vi "Main.vi"() -> ()   [LabVIEW 2018, in "Personalities Tool.lvlib"]
uses:
  Personalities Tool.lvlib
  Controls/QMH Data.ctl
  Controls/Personality Type.ctl
  Controls/roboRIO Connection Information.ctl
  Controls/Diff Key.ctl
  subVIs/Message Queue/Enqueue Message (Single).vi
panel:
  out "Personality":string
  out "Status":string
  in  "File editor":string
  in  "Download personality to RIO":bool
  in  "Save personality locally":bool
  in  "Connect":bool
  in  "Open local personality":bool
  in  "Stop":bool
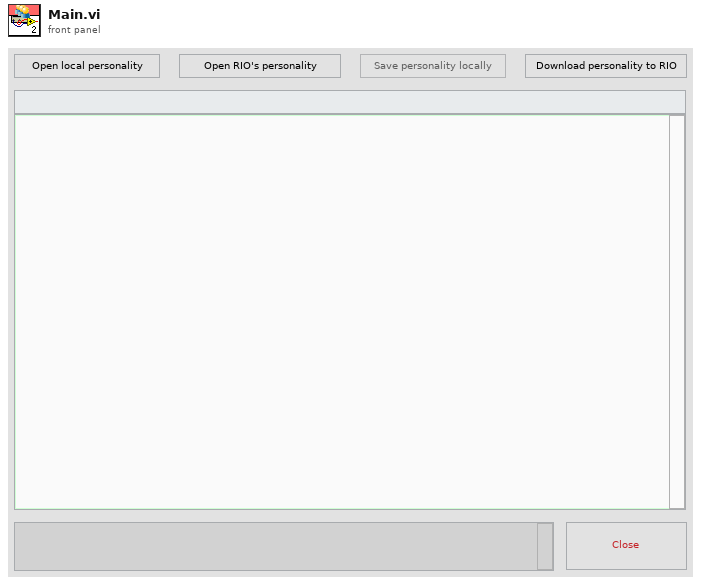
[diagram p1: front panel]
types:
  T1 = typedef "Personalities Tool.lvlib/QMH Data.ctl" = cluster{"Status":string, "Open Personality File Path":path, "File text":string, "Selected Personality":T2, "roboRIO Connection Information":T3, "VI reference":refnum<vi>, "Save personality locally reference":refnum<vi>, "File editor reference":refnum<vi>}
  T2 = typedef "Personalities Tool.lvlib/Personality Type.ctl" = cluster{"Valid personality?":bool, "Personality":string}
  T3 = typedef "Personalities Tool.lvlib/roboRIO Connection Information.ctl" = cluster{"Connected?":bool, "IP Address":string, "SN":string, "Personality":T2, "Name":string}
  T4 = typedef "Personalities Tool.lvlib/All Message Queues.ctl" = cluster{"UI":refnum<queue>}
  T5 = enum8{"Enabled", "Disabled", "Disabled and Grayed Out"}
  T6 = typedef "Personalities Tool.lvlib/Diff Key.ctl" = cluster{"Section":string, "Local":variant, "roboRIO":variant, "Selection":enum32{"Item 0", "Item 1"}, "Key":string}
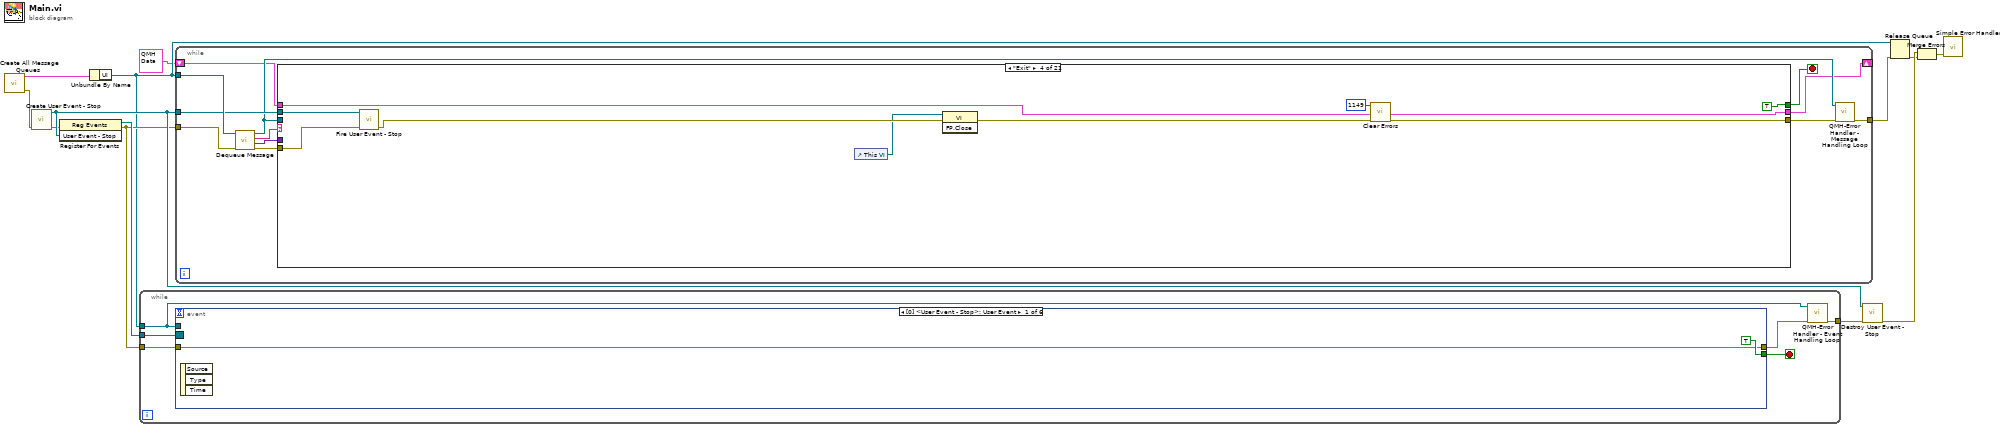
[diagram p0: block diagram]
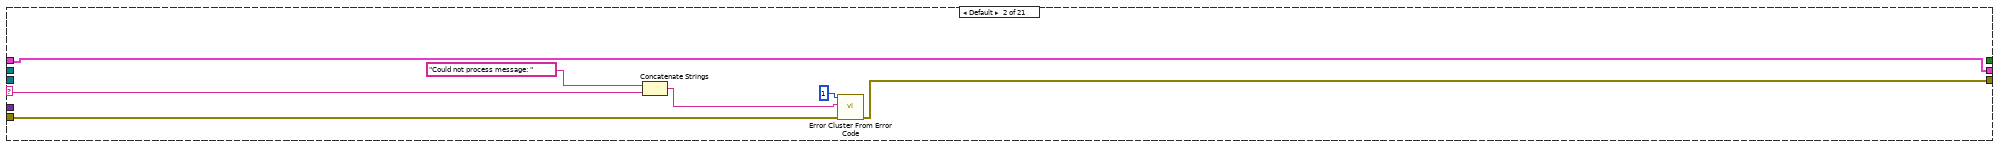
[diagram p3: hidden frame]
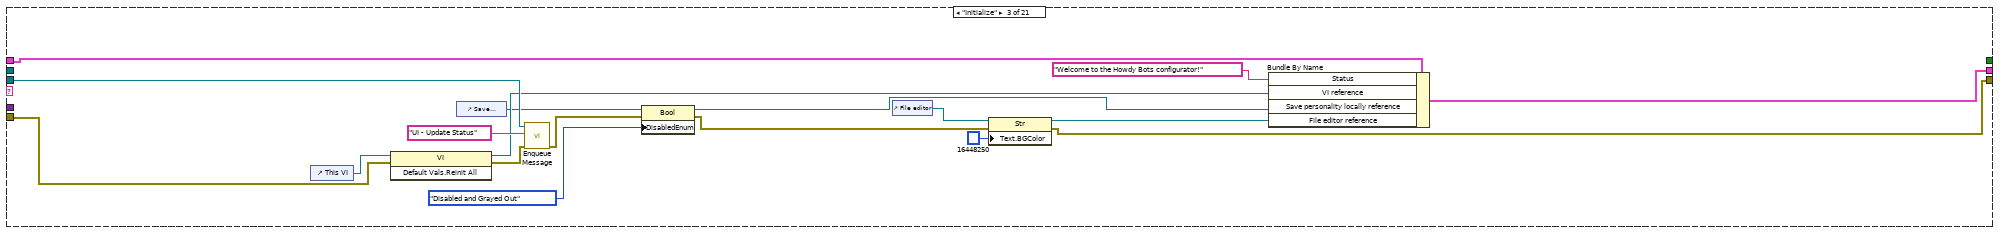
[diagram p4: hidden frame]
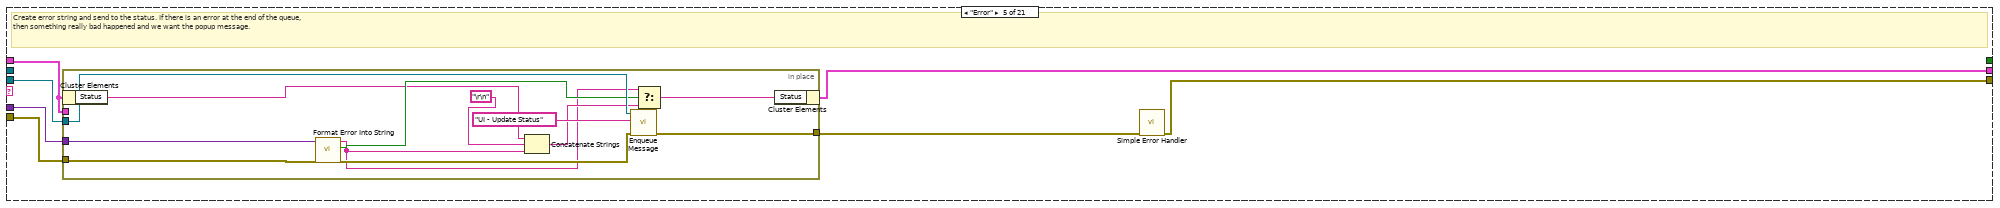
[diagram p5: hidden frame]
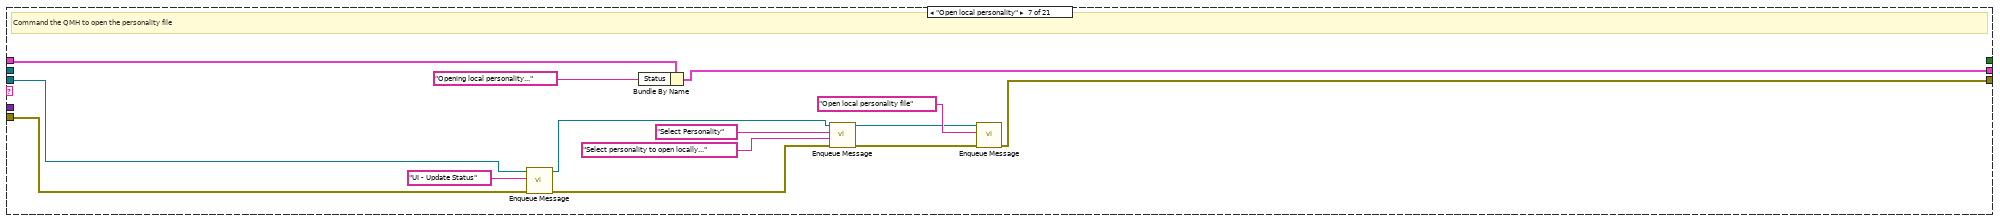
[diagram p7: hidden frame]
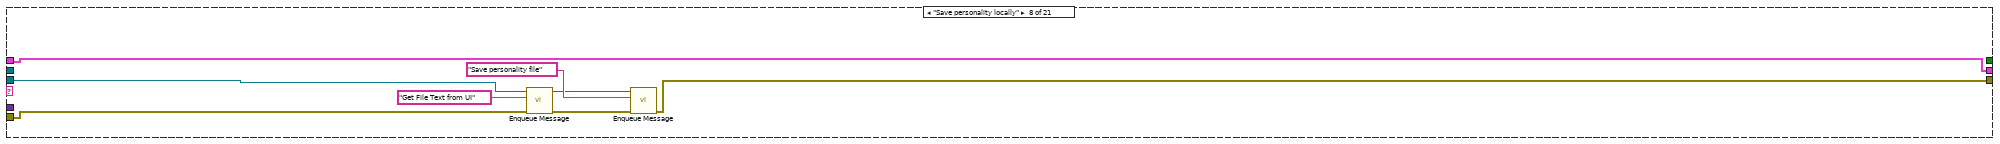
[diagram p8: hidden frame]
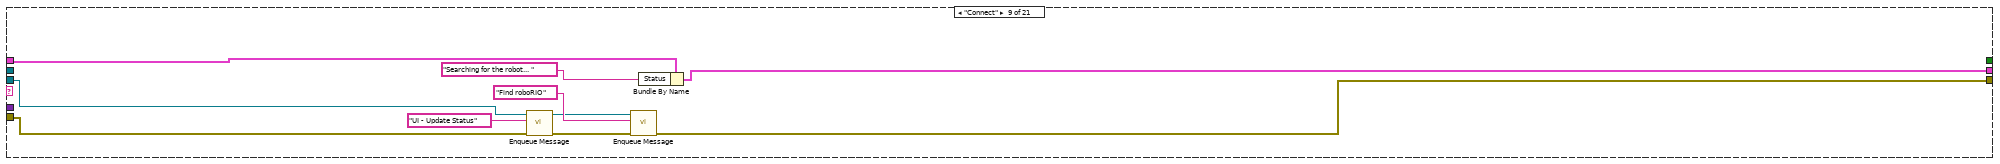
[diagram p9: hidden frame]
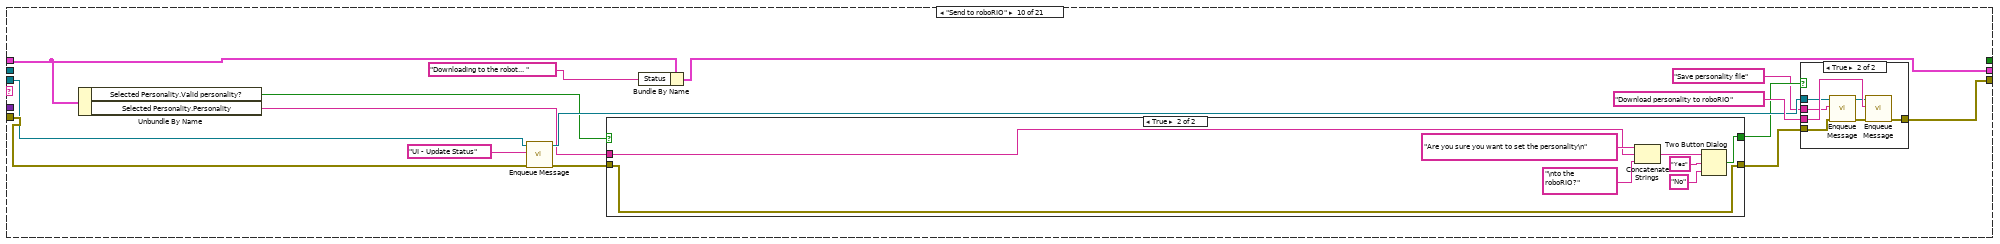
[diagram p10: hidden frame]
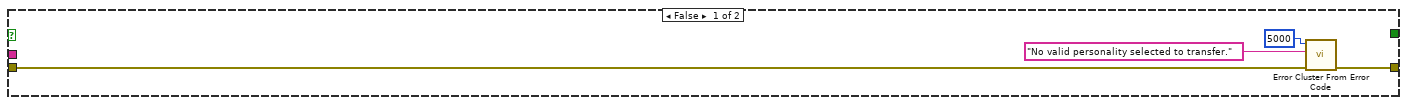
[diagram p11: hidden frame]
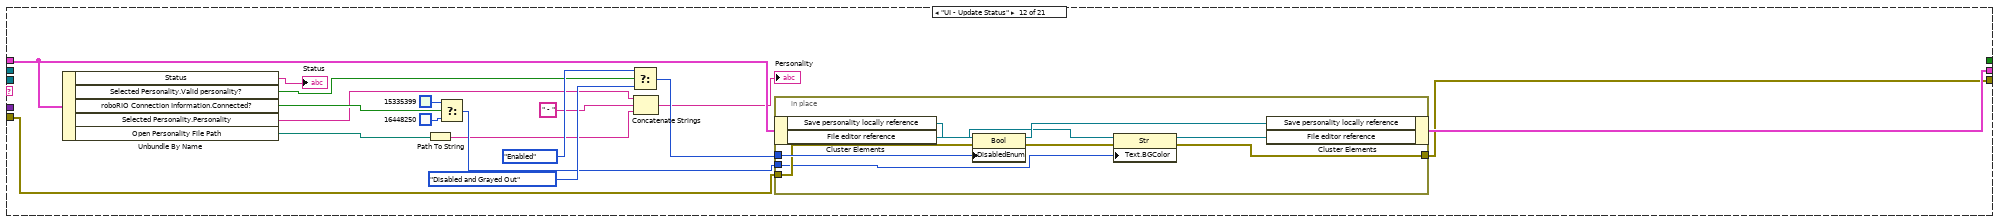
[diagram p14: hidden frame]
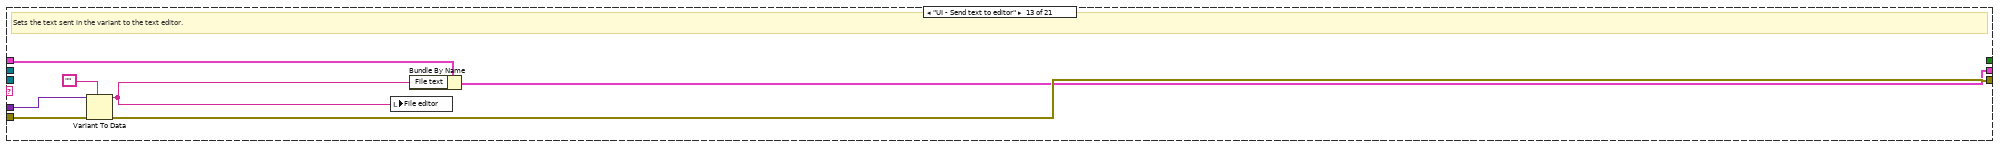
[diagram p15: hidden frame]
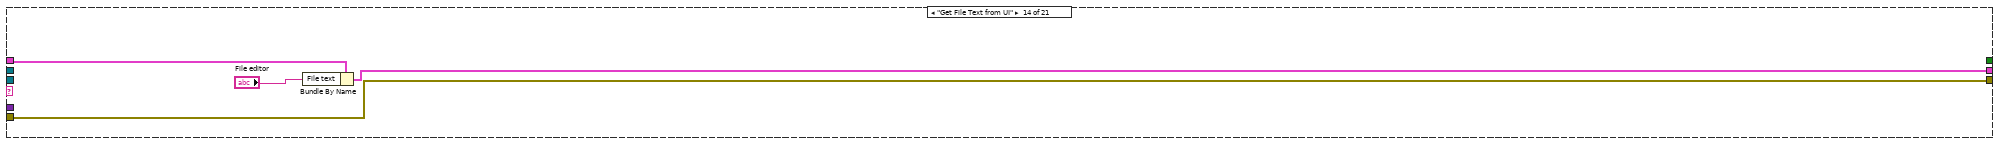
[diagram p16: hidden frame]
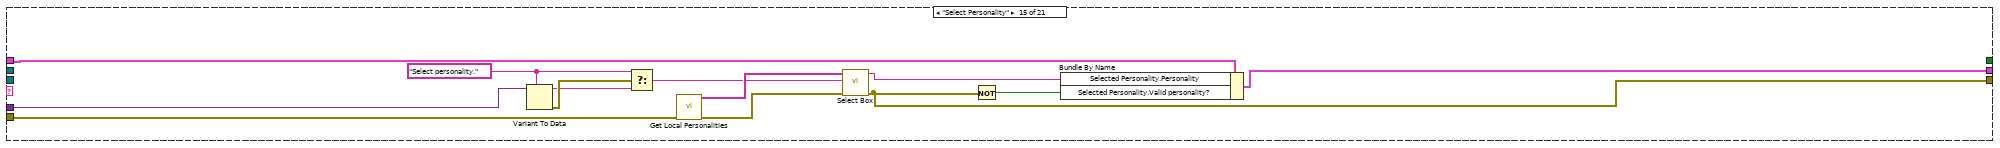
[diagram p17: hidden frame]
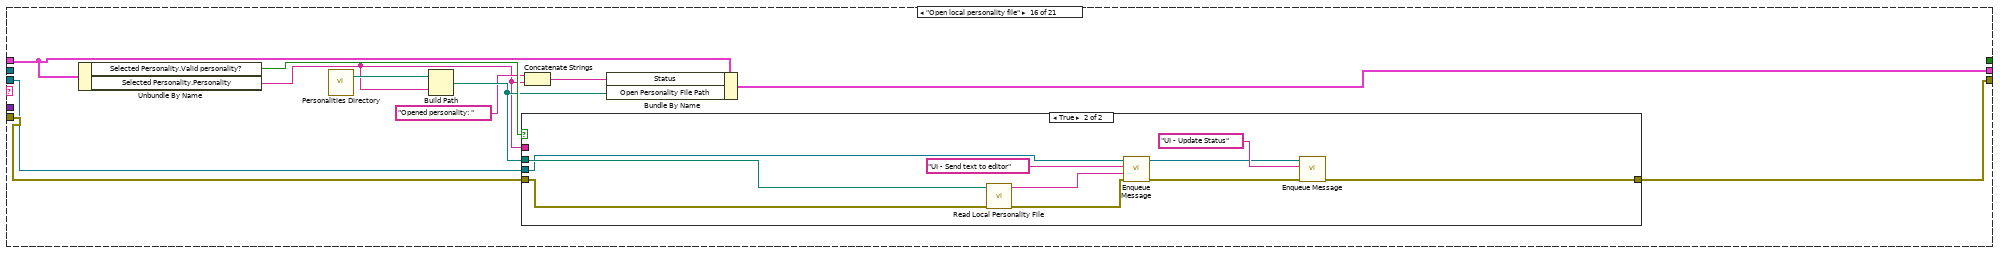
[diagram p18: hidden frame]
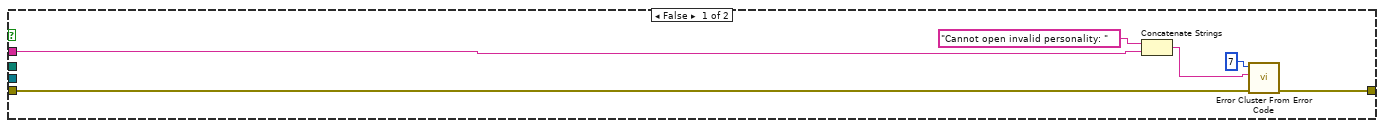
[diagram p19: hidden frame]
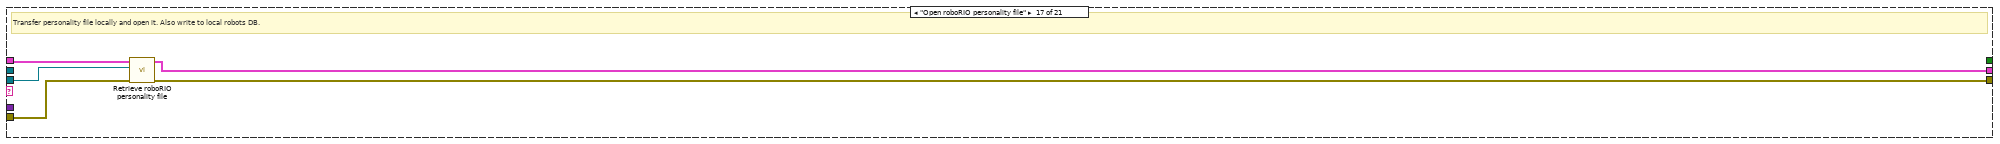
[diagram p20: hidden frame]
diagram:
  n1 = call "Create All Message Queues.vi"() -> ("error out"=w10:errorcluster, "Message Queues out"=w11:T4)  [unwired: 10 in]
  n2 = call "Create User Event - Stop.vi"("error in (no error)"=w10) -> ("error out"=w9:errorcluster, "User Event - Stop"=w12:refnum<user-event>)  [unwired: 9 in]
  n3 = register-events(error in=w9, w12) -> (reference out=w13:refnum<event-registration>, error out=w8:errorcluster)  [unwired: 1 in]
  n4 = Unbundle By Name(w11) -> ("UI"=w4:refnum<queue>)
  n5 = while {
    tunnel: w13 -> [w19]
    tunnel: w4 -> [w14]
    tunnel: w8 -> [w18]
    tunnel: [w15] -> w7
    stop <- w17 stop-if-true
    n6 = event shown="[0] <User Event - Stop>: User Event" {
      selector: w19 -> [_ _ _ _ _ _]
      dyn-events: _ -> [_ _ _ _ _ _]
      timeout: _ -> [_ _ _ _ _ _]
      tunnel: w14 -> [_ w22 w37 w41 w45 w52]
      tunnel: w18 -> [w20 w24 w39 w43 w47 w50]
      tunnel: [TRUE _ _ _ _ _] -> w17
      tunnel: [w20 w27 w38 w42 w46 w54] -> w16
      event User Event {
        n7 = event-data() -> ()  [unwired: 1 in, 3 out]
      }
      event "Stop": Value Change; Panel Close {
        n8 = event-data() -> ()  [unwired: 1 in, 3 out]
        n9 = disable-structure shown="Enabled" {
          disable-tunnel: [w28 _] -> w25
          frame Disabled {
            n10 = Two Button Dialog(message="Save opened personality before closing?", 1:"No" ("F button name (\"Cancel\")"), 2:"Yes" ("T button name (\"OK\")")) -> (T button?=w28:bool)
          }
          frame Enabled {
            # "Disabled saving check to ensure we do not accidentally override the\nfile with constants and introduce typos"
          }
        }
        n11 = case shown="True" w25 {
          tunnel: [w32 w34] -> w23
          tunnel: w24 -> [w32 w35]
          tunnel: w22 -> [_ w33]
          frame False {
          }
          frame True {
            n12 = call-poly "Enqueue Message.vi"("error in (no error)"=w35, "Message"="Save personality locally", "Message Queue"=w33) -> ("error out"=w34:errorcluster)  [unwired: 7 in, 1 out]
          }
        }
        n13 = call-poly "Enqueue Message.vi"("error in (no error)"=w23, "Message"="Exit", "Message Queue"=w22) -> ("error out"=w27:errorcluster)  [unwired: 7 in, 1 out]
      }
      event "Open local personality": Value Change {
        n14 = event-data() -> ()  [unwired: 1 in, 3 out]
        n15 = call-poly "Enqueue Message.vi"("error in (no error)"=w39, "Message"="Open local personality", "Message Queue"=w37) -> ("error out"=w38:errorcluster)  [unwired: 7 in, 1 out]
      }
      event "Connect": Value Change {
        n16 = event-data() -> ()  [unwired: 1 in, 3 out]
        n17 = call-poly "Enqueue Message.vi"("error in (no error)"=w43, "Message"="Connect", "Message Queue"=w41) -> ("error out"=w42:errorcluster)  [unwired: 7 in, 1 out]
      }
      event "Save personality locally": Value Change {
        n18 = event-data() -> ()  [unwired: 1 in, 3 out]
        n19 = call-poly "Enqueue Message.vi"("error in (no error)"=w47, "Message"="Save personality locally", "Message Queue"=w45) -> ("error out"=w46:errorcluster)  [unwired: 7 in, 1 out]
      }
      event "Download personality to RIO": Value Change {
        n20 = event-data() -> ()  [unwired: 1 in, 3 out]
        n21 = call-poly "Enqueue Message.vi"("error in (no error)"=w50, "Message"="Save personality locally", "Message Queue"=w52) -> ("error out"=w49:errorcluster, "dup Message Queue"=w51:refnum<queue>)  [unwired: 7 in]
        n22 = call-poly "Enqueue Message.vi"("error in (no error)"=w49, "Message"="Send to roboRIO", "Message Queue"=w51) -> ("error out"=w54:errorcluster)  [unwired: 7 in, 1 out]
      }
    }
    n23 = call "QMH-Error Handler - Event Handling Loop.vi"("error in (no error)"=w16, "Message Queue"=w14) -> ("dup error in"=w15:errorcluster)  [unwired: 8 in, 1 out]
  }
  n24 = while {
    tunnel: w12 -> [w60]
    tunnel: w4 -> [w67]
    tunnel: w8 -> [w66]
    tunnel: [w61] -> w5
    shift-right: [w57] -> _
    shift-left: T1 {"Status"="", "Open Personality File Path"=path "", "File text"="", "Selected Personality"={"Valid personality?"=FALSE, "Personality"=""}, "roboRIO Connection Information"={"Connected?"=FALSE, "IP Address"="", "SN"="", "Personality"={"Valid personality?"=FALSE, "Personality"=""}, "Name"=""}, "VI reference"=refnum, "Save personality locally reference"=refnum, "File editor reference"=refnum} ("UI Data") -> [w56]
    stop <- w58 stop-if-true
    n25 = call "Dequeue Message.vi"("error in (no error)"=w66, "Message Queue"=w67) -> ("error out"=w64:errorcluster, "Message Data"=w63:variant, "Message"=w65:string, "dup Message Queue"=w59:refnum<queue>)  [unwired: 6 in]
    n26 = case shown="\"Exit\"" w65 {
      selector: w65 -> [_ w71 _ _ _ _ _ _ _ _ _ _ _ _ _ _ _ _ _ _ _]
      tunnel: w64 -> [w68 w76 w87 w103 w110 w123 w135 w141 w151 w168 w192 w203 w226 w230 w239 w253 w275 w285 w311 w328 w350]
      tunnel: [w68 w75 w80 w96 w106 w123 w126 w139 w149 w166 w192 w204 w225 w230 w241 w251 w276 w283 w312 w314 w347] -> w62
      tunnel: w63 -> [_ _ _ _ w109 _ _ _ _ _ _ _ w224 _ w236 _ _ _ _ _ w349]
      tunnel: w59 -> [_ _ w90 _ w108 _ w136 w140 w150 w167 _ _ _ _ _ w248 w272 w282 w309 w316 w341]
      tunnel: w60 -> [_ _ _ w102 _ _ _ _ _ _ _ _ _ _ _ _ _ _ _ _ _]
      tunnel: [_ _ _ TRUE _ _ _ _ _ _ _ _ _ _ _ _ _ _ _ _ _] -> w58
      tunnel: [w69 w70 w93 w99 w104 w124 w134 w146 w148 w165 w193 w209 w222 w229 w243 w254 w274 w286 w313 w322 w345] -> w57
      tunnel: w56 -> [w69 w70 w94 w99 w105 w124 w138 w146 w156 w162 w193 w210 w227 w231 w244 w255 w273 w287 w310 w327 w342]
      frame "---BASE QMH MESSAGES---" {
        # "This case must not execute ever, used just for documentation"
      }
      frame Default {
        n27 = Concatenate Strings("Could not process message: " ("error message (\"\")"), w71) -> (w72:string)
        n28 = call <vilib>:"Error Cluster From Error Code.vi"("error in (no error)"=w76, "error message (\"\")"=w72, "error code (0)"=1) -> ("error out"=w75:errorcluster)  [unwired: 6 in]
      }
      frame "Initialize" {
        n29 = control-ref of="This VI"() -> (w88:refnum<vi>)
        n30 = invoke class="VI" method="Default Vals.Reinit All"(reference=w88, error in=w87) -> (reference out=w85:refnum<vi>, error out=w86:errorcluster)  [unwired: 1 in, 1 out]
        n31 = control-ref of="Save personality locally"() -> (w83:refnum<vi>)
        n32 = call-poly "Enqueue Message.vi"("error in (no error)"=w86, "Message"="UI - Update Status", "Message Queue"=w90) -> ("error out"=w89:errorcluster)  [unwired: 7 in, 1 out]
        n33 = property class="Bool"(reference=w83, error in=w89, "DisabledEnum"=T5."Disabled and Grayed Out" ("Disabled")) -> (reference out=w82:refnum<vi>, error out=w84:errorcluster)
        n34 = control-ref of="File editor"() -> (w79:refnum<vi>)
        n35 = property class="Str"(reference=w79, error in=w84, "Text.BGColor"=u32 16448250 ("Text.Colors:BG Color")) -> (reference out=w78:refnum<vi>, error out=w80:errorcluster)
        n36 = Bundle By Name(cluster=w94, "Status"="Welcome to the Howdy Bots configurator!" ("element"), "VI reference"=w85, "Save personality locally reference"=w82, "File editor reference"=w78) -> (w93:T1)
      }
      frame "Exit" {
        n37 = call "Fire User Event - Stop.vi"("error in (no error)"=w103, "User Event - Stop"=w102) -> ("error out"=w101:errorcluster)  [unwired: 9 in]
        n38 = control-ref of="This VI"() -> (w97:refnum<vi>)
        n39 = invoke class="VI" method="FP.Close"(reference=w97, error in=w101) -> (error out=w98:errorcluster)  [unwired: 1 in, 2 out]
        n40 = call <vilib>:"Clear Errors.vi"("error in (no error)"=w98, "specific error code to clear (0: all)"=1149) -> ("error out"=w96:errorcluster)  [unwired: 4 in, 1 out]
      }
      frame "Error" {
        # "Create error string and send to the status. If there is an error at the end of the queue, \nthen something really bad happened and we want the popup message."
        n41 = in-place {
          in-place-border: w110 -> [w122]
          in-place-border: w109 -> [w121]
          in-place-border: w108 -> [w120]
          in-place-border: [w118] -> w107
          in-place-border: w105 -> [_]
          n42 = in-place-cluster #1(w105) -> ("Status"=w112:string)
          n43 = call "Format Error Into String.vi"("error in (no error)"=w122, "Message Data"=w121) -> ("error out"=w117:errorcluster, "error?"=w116:bool, "message"=w114:string)  [unwired: 7 in]
          n44 = Concatenate Strings(w112, "\r\n", w114) -> (w115:string)
          n45 = call-poly "Enqueue Message.vi"("error in (no error)"=w117, "Message"="UI - Update Status", "Message Queue"=w120) -> ("error out"=w118:errorcluster)  [unwired: 7 in, 1 out]
          n46 = Select(t=w114, s=w116, f=w115) -> (s? t:f=w111:string)
          n47 = in-place-cluster #1("Status"=w111) -> (w104:T1)
        }
        n48 = call <vilib>:"Simple Error Handler.vi"("error in (no error)"=w107) -> ("error out"=w106:errorcluster)  [unwired: 4 in, 4 out]
      }
      frame "---UI MESSAGES---" {
        # "This case must not execute ever, used just for documentation"
      }
      frame "Open local personality" {
        # "Command the QMH to open the personality file"
        n49 = call-poly "Enqueue Message.vi"("error in (no error)"=w135, "Message"="UI - Update Status", "Message Queue"=w136) -> ("error out"=w130:errorcluster, "dup Message Queue"=w131:refnum<queue>)  [unwired: 7 in]
        n50 = Bundle By Name(cluster=w138, "Status"="Opening local personality...") -> (w134:T1)
        n51 = call-poly "Enqueue Message.vi"("error in (no error)"=w130, "Message Data"="Select personality to open locally..." ("Message"), "Message"="Select Personality", "Message Queue"=w131) -> ("error out"=w127:errorcluster, "dup Message Queue"=w125:refnum<queue>)  [unwired: 6 in]
        n52 = call-poly "Enqueue Message.vi"("error in (no error)"=w127, "Message"="Open local personality file", "Message Queue"=w125) -> ("error out"=w126:errorcluster)  [unwired: 7 in, 1 out]
      }
      frame "Save personality locally" {
        n53 = call-poly "Enqueue Message.vi"("error in (no error)"=w141, "Message"="Get File Text from UI", "Message Queue"=w140) -> ("error out"=w142:errorcluster, "dup Message Queue"=w143:refnum<queue>)  [unwired: 7 in]
        n54 = call-poly "Enqueue Message.vi"("error in (no error)"=w142, "Message"="Save personality file", "Message Queue"=w143) -> ("error out"=w139:errorcluster)  [unwired: 7 in, 1 out]
      }
      frame "Connect" {
        n55 = call-poly "Enqueue Message.vi"("error in (no error)"=w151, "Message"="UI - Update Status", "Message Queue"=w150) -> ("error out"=w152:errorcluster, "dup Message Queue"=w153:refnum<queue>)  [unwired: 7 in]
        n56 = call-poly "Enqueue Message.vi"("error in (no error)"=w152, "Message"="Find roboRIO", "Message Queue"=w153) -> ("error out"=w149:errorcluster)  [unwired: 7 in, 1 out]
        n57 = Bundle By Name(cluster=w156, "Status"="Searching for the robot... ") -> (w148:T1)
      }
      frame "Send to roboRIO" {
        n58 = Unbundle By Name(w162) -> ("Selected Personality.Valid personality?"=w160:bool, "Selected Personality.Personality"=w161:string)
        n59 = call-poly "Enqueue Message.vi"("error in (no error)"=w168, "Message"="UI - Update Status", "Message Queue"=w167) -> ("error out"=w159:errorcluster, "dup Message Queue"=w169:refnum<queue>)  [unwired: 7 in]
        n60 = case shown="True" w160 {
          tunnel: [_ w180] -> w163
          tunnel: w161 -> [_ w177]
          tunnel: [w174 w176] -> w158
          tunnel: w159 -> [w175 w176]
          frame False {
            n61 = call <vilib>:"Error Cluster From Error Code.vi"("error in (no error)"=w175, "error message (\"\")"="No valid personality selected to transfer." ("error message (\"\")"), "error code (0)"=5000) -> ("error out"=w174:errorcluster)  [unwired: 6 in]
          }
          frame True {
            n62 = Concatenate Strings("Are you sure you want to set the personality\n" ("message"), w177, "\nto the roboRIO?" ("message")) -> (w179:string)
            n63 = Two Button Dialog(message=w179, 1:"No" ("F button name (\"Cancel\")"), 2:"Yes" ("T button name (\"OK\")")) -> (T button?=w180:bool)
          }
        }
        n64 = Bundle By Name(cluster=w162, "Status"="Downloading to the robot... ") -> (w165:T1)
        n65 = case shown="True" w163 {
          tunnel: "Download personality to roboRIO" ("Message") -> [_ w191]
          tunnel: w169 -> [_ w187]
          tunnel: w158 -> [w184 w190]
          tunnel: [w184 w188] -> w166
          tunnel: "Save personality file" ("Message") -> [_ w185]
          frame False {
          }
          frame True {
            n66 = call-poly "Enqueue Message.vi"("error in (no error)"=w190, "Message"=w185, "Message Queue"=w187) -> ("error out"=w189:errorcluster, "dup Message Queue"=w186:refnum<queue>)  [unwired: 7 in]
            n67 = call-poly "Enqueue Message.vi"("error in (no error)"=w189, "Message"=w191, "Message Queue"=w186) -> ("error out"=w188:errorcluster)  [unwired: 7 in, 1 out]
          }
        }
      }
      frame "---SUPPORT FUNCTIONS---" {
        # "This case must not execute ever, used just for documentation"
      }
      frame "UI - Update Status" {
        n68 = Unbundle By Name(w210) -> ("Status"=→"Status":string, "Selected Personality.Valid personality?"=w206:bool, "roboRIO Connection Information.Connected?"=w202:bool, "Selected Personality.Personality"=w197:string, "Open Personality File Path"=w198:path)
        n69 = Path To String(path=w198) -> (string=w196:string)
        n70 = Select(t=u32 15335399 ("Text.Colors:FG Color"), s=w202, f=u32 16448250 ("Text.Colors:BG Color")) -> (s? t:f=w201:u32)
        n71 = Select(t=T5."Enabled" ("Disabled"), s=w206, f=T5."Disabled and Grayed Out" ("Disabled")) -> (s? t:f=w207:T5)
        n72 = Concatenate Strings(w197, " - " ("string"), w196) -> (→"Personality":string)
        n73 = in-place {
          in-place-border: w207 -> [w220]
          in-place-border: w203 -> [w217]
          in-place-border: [w213] -> w204
          in-place-border: w201 -> [w212]
          n74 = in-place-cluster #2(w210) -> ("Save personality locally reference"=w219:refnum<vi>, "File editor reference"=w216:refnum<vi>)
          n75 = property class="Bool"(reference=w219, error in=w217, "DisabledEnum"=w220) -> (reference out=w218:refnum<vi>, error out=w214:errorcluster)
          n76 = property class="Str"(reference=w216, error in=w214, "Text.BGColor"=w212) -> (reference out=w215:refnum<vi>, error out=w213:errorcluster)
          n77 = in-place-cluster #2("Save personality locally reference"=w218, "File editor reference"=w215) -> (w209:T1)
        }
      }
      frame "UI - Send text to editor" {
        # "Sets the text sent in the variant to the text editor."
        n78 = Variant To Data(error in=w226, type="", Variant=w224) -> (data=w221:string, error out=w225:errorcluster)
        n79 = local write "File editor"(w221) -> ()
        n80 = Bundle By Name(cluster=w227, "File text"=w221) -> (w222:T1)
      }
      frame "Get File Text from UI" {
        n81 = Bundle By Name(cluster=w231, "File text"="File editor") -> (w229:T1)
      }
      frame "Select Personality" {
        w234 = "Select personality."
        n82 = Variant To Data(type=w234, Variant=w236) -> (data=w233:string, error out=w235:errorcluster)  [unwired: 1 in]
        n83 = Select(t=w234, s=w235, f=w233) -> (s? t:f=w232:string)
        n84 = call "Get Local Personalities.vi"("error in (no error)"=w239) -> ("error out"=w238:errorcluster, "Personalities"=w237:string[])  [unwired: 9 in]
        n85 = call "Select Box.vi"("error in (no error)"=w238, "UI message"=w232, "Selections available"=w237) -> ("error out"=w241:errorcluster, "Selection"=w242:string)  [unwired: 7 in]
        n86 = Not(x=w241) -> (.not. x?=w240:bool)
        n87 = Bundle By Name(cluster=w244, "Selected Personality.Personality"=w242, "Selected Personality.Valid personality?"=w240) -> (w243:T1)
      }
      frame "Open local personality file" {
        n88 = Unbundle By Name(w255) -> ("Selected Personality.Valid personality?"=w252:bool, "Selected Personality.Personality"=w245:string)
        n89 = call "Personalities Directory.vi"() -> ("appended path"=w250:path)  [unwired: 3 in]
        n90 = Build Path(base path=w250, name or relative path=w245) -> (appended path=w249:path)
        n91 = case shown="True" w252 {
          tunnel: w253 -> [w261 w271]
          tunnel: w245 -> [w256 _]
          tunnel: [w260 w262] -> w251
          tunnel: w249 -> [_ w270]
          tunnel: w248 -> [_ w267]
          frame False {
            n92 = Concatenate Strings("Cannot open invalid personality: " ("error message (\"\")"), w256) -> (w257:string)
            n93 = call <vilib>:"Error Cluster From Error Code.vi"("error in (no error)"=w261, "error message (\"\")"=w257, "error code (0)"=7) -> ("error out"=w260:errorcluster)  [unwired: 6 in]
          }
          frame True {
            n94 = call "Read Local Personality File.vi"("error in (no error)"=w271, "File Path"=w270) -> ("error out"=w268:errorcluster, "Personality text"=w266:string)  [unwired: 7 in, 1 out]
            n95 = call-poly "Enqueue Message.vi"("error in (no error)"=w268, "Message Data"=w266, "Message"="UI - Send text to editor", "Message Queue"=w267) -> ("error out"=w263:errorcluster, "dup Message Queue"=w264:refnum<queue>)  [unwired: 6 in]
            n96 = call-poly "Enqueue Message.vi"("error in (no error)"=w263, "Message"="UI - Update Status", "Message Queue"=w264) -> ("error out"=w262:errorcluster)  [unwired: 7 in, 1 out]
          }
        }
        n97 = Concatenate Strings("Opened personality: " ("Status"), w245) -> (w246:string)
        n98 = Bundle By Name(cluster=w255, "Status"=w246, "Open Personality File Path"=w249) -> (w254:T1)
      }
      frame "Open roboRIO personality file" {
        # "Transfer personality file locally and open it. Also write to local robots DB."
        n99 = call "Retrieve roboRIO personality file.vi"("error in (no error)"=w275, "Message Queue"=w272, "UI Data Out"=w273) -> ("error out"=w276:errorcluster, "UI Data in"=w274:T1)  [unwired: 7 in]
      }
      frame "Save personality file" {
        n100 = Unbundle By Name(w287) -> ("Selected Personality.Valid personality?"=w284:bool, "Selected Personality.Personality"=w281:string, "Open Personality File Path"=w280:path, "File text"=w279:string)
        n101 = case shown="False" w284 {
          tunnel: w285 -> [w294 w305]
          tunnel: w281 -> [w291 w297]
          tunnel: [w293 w296] -> w283
          tunnel: w280 -> [w288 w306]
          tunnel: w282 -> [_ w308]
          tunnel: [w289 w298] -> w278
          tunnel: w279 -> [_ w299]
          tunnel: [w288 w295] -> w277
          frame False {
            n102 = Concatenate Strings("Cannot save invalid personality: " ("error message (\"\")"), w291) -> (w289:string)
            n103 = call <vilib>:"Error Cluster From Error Code.vi"("error in (no error)"=w294, "error message (\"\")"=w289, "error code (0)"=7) -> ("error out"=w293:errorcluster)  [unwired: 6 in]
          }
          frame True {
            n104 = call "Save Local Personality File.vi"("error in (no error)"=w305, "New Content"=w299, "File Path"=w306) -> ("error out"=w300:errorcluster, "Path out"=w295:path)  [unwired: 7 in]
            n105 = call-poly "Enqueue Message.vi"("Message"="UI - Update Status", "Message Queue"=w308) -> ("error out"=w301:errorcluster)  [unwired: 8 in, 1 out]
            n106 = Merge Errors(w300, w301) -> (w296:errorcluster)
            n107 = Select(t="Could not save personality: ", s=w296, f="Saved personality: " ("Status")) -> (s? t:f=w304:string)
            n108 = Concatenate Strings(w304, w297) -> (w298:string)
          }
        }
        n109 = Bundle By Name(cluster=w287, "Open Personality File Path"=w277, "Status"=w278) -> (w286:T1)
      }
      frame "Find roboRIO" {
        n110 = call "Find roboRIO.vi"("error in (no error)"=w311, "Queue In"=w309, "UI Data in"=w310) -> ("error out"=w312:errorcluster, "UI Data out"=w313:T1)  [unwired: 7 in]
      }
      frame "Download personality to roboRIO" {
        # "#TODO"
        n111 = Unbundle By Name(w327) -> ("Open Personality File Path"=w318:path, "roboRIO Connection Information"=w326:T3)
        n112 = call "Transfer file to roboRIO.vi"("error in (no error)"=w328, "roboRIO Connection Information in"=w326, "Configuration File Path"=w318) -> ("error out"=w325:errorcluster, "roboRIO Connection Information out"=w324:T3, "Status"=w323:string)  [unwired: 6 in]
        n113 = case shown="Error" w325 {
          selector: w325 -> [w331 _]
          tunnel: [w331 w335] -> w320
          tunnel: [w330 w333] -> w319
          tunnel: w324 -> [w330 _]
          tunnel: [w329 w334] -> w321
          tunnel: w323 -> [w329 _]
          tunnel: w318 -> [_ w332]
          frame No Error {
          }
          frame Error {
            # "If we are already connected, \nwe try that connection the first time.\nIf we fail, then we query for roboRIOs again"
            n114 = call "Transfer file to roboRIO.vi"("Configuration File Path"=w332) -> ("error out"=w335:errorcluster, "roboRIO Connection Information out"=w333:T3, "Status"=w334:string)  [unwired: 8 in]
          }
        }
        n115 = Bundle By Name(cluster=w327, "Status"=w321, "roboRIO Connection Information"=w319) -> (w322:T1)
        n116 = call "Set Personality with SN.vi"("error in (no error)"=w320, "roboRIO Connection Information"=w319) -> ("error out"=w315:errorcluster)  [unwired: 9 in]
        n117 = call-poly "Enqueue Message.vi"("error in (no error)"=w315, "Message"="UI - Update Status", "Message Queue"=w316) -> ("error out"=w314:errorcluster)  [unwired: 7 in, 1 out]
      }
      frame "Diff" {
        n118 = Bundle("Diff conflicts"=T6[] [], path[] []) -> (w339:cluster{"Diff conflicts":T6[], path[]})  [unwired: 1 in]
        n119 = Variant To Data(error in=w350, type=w339, Variant=w349) -> (data=w346:cluster{"Diff conflicts":T6[], path[]}, error out=w348:errorcluster)
        n120 = Unbundle(w346) -> ("Diff conflicts"=w336:T6[], w338:path[])
        n121 = Index Array(array=w338) -> (element #1=w343:path, element #2=w344:path)  [unwired: 2 in]
        n122 = call "Diff Tool.vi"("Diff conflicts"=w336, "Message Queue"=w341, "error in (no error)"=w348, "roboRIO"=w344, "Local"=w343, "UI Data in"=w342) -> ("error out"=w347:errorcluster, "UI Data out"=w345:T1)  [unwired: 4 in]
      }
    }
    n123 = call "QMH-Error Handler - Message Handling Loop.vi"("error in (no error)"=w62, "Message Queue"=w59) -> ("dup error in"=w61:errorcluster)  [unwired: 8 in, 1 out]
  }
  n124 = call "Destroy User Event - Stop.vi"("error in (no error)"=w7, "User Event - Stop"=w12) -> ("error out"=w6:errorcluster)  [unwired: 9 in]
  n125 = Release Queue(queue=w4, error in (no error)=w5) -> (error out=w3:errorcluster)  [unwired: 1 in, 2 out]
  n126 = Merge Errors(w6, w3) -> (w2:errorcluster)
  n127 = call <vilib>:"Simple Error Handler.vi"("error in (no error)"=w2) -> ()  [unwired: 4 in, 5 out]
